vi "VI to JSON Graph Descr.vi"(8 "error in (no error)":errorcluster, 11 "vi path":path) -> (0 "error out":errorcluster, 1 "# of Refs":i32, 2 "Objects with owner":T2[](array[typedef]) {"Ownder_UID" format="%x"; "UID" format="%x"; "ClassID" format="%x"})   [LabVIEW 2020]
uses:
  ObjDescription.ctl
  Wire_Source_and_Sinks_IDs.ctl
  <vilib>/Utility/traverseref.llb/TRef TravTarget.ctl
  <vilib>/Utility/traverseref.llb/VI Scripting - Traverse.lvlib
panel:
  out "Wires":T1[](array[typedef])
  in  "Traverse Generated Code (F)":bool
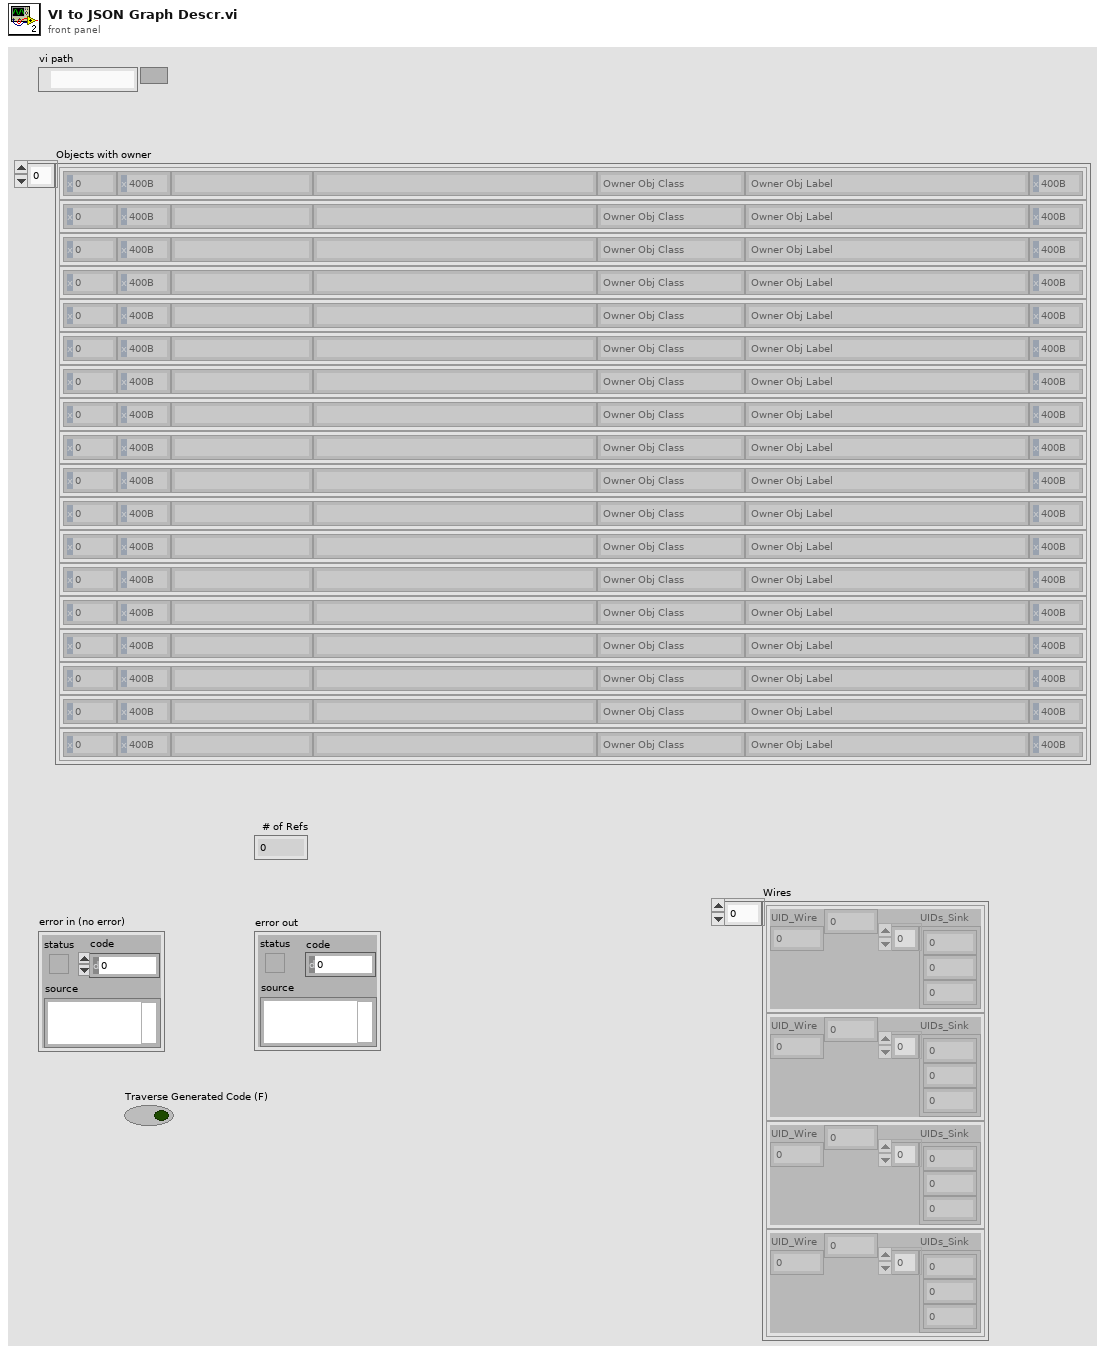
[diagram p1: front panel]
types:
  T1 = typedef "Wire_Source_and_Sinks_IDs.ctl" = cluster{"UID_Wire":i32, "UID_Source":i32, "UIDs_Sink":i32[]}
  T2 = typedef "ObjDescription.ctl" = cluster{"ClassID":u32, "UID":u32, "ClassName":string, "LabelText":string, "OwnerClass":string, "OwnerName":string, "Ownder_UID":u32}
  T3 = typedef "TRef TravTarget.ctl" = enum16{"FP", "BD", "Other"}
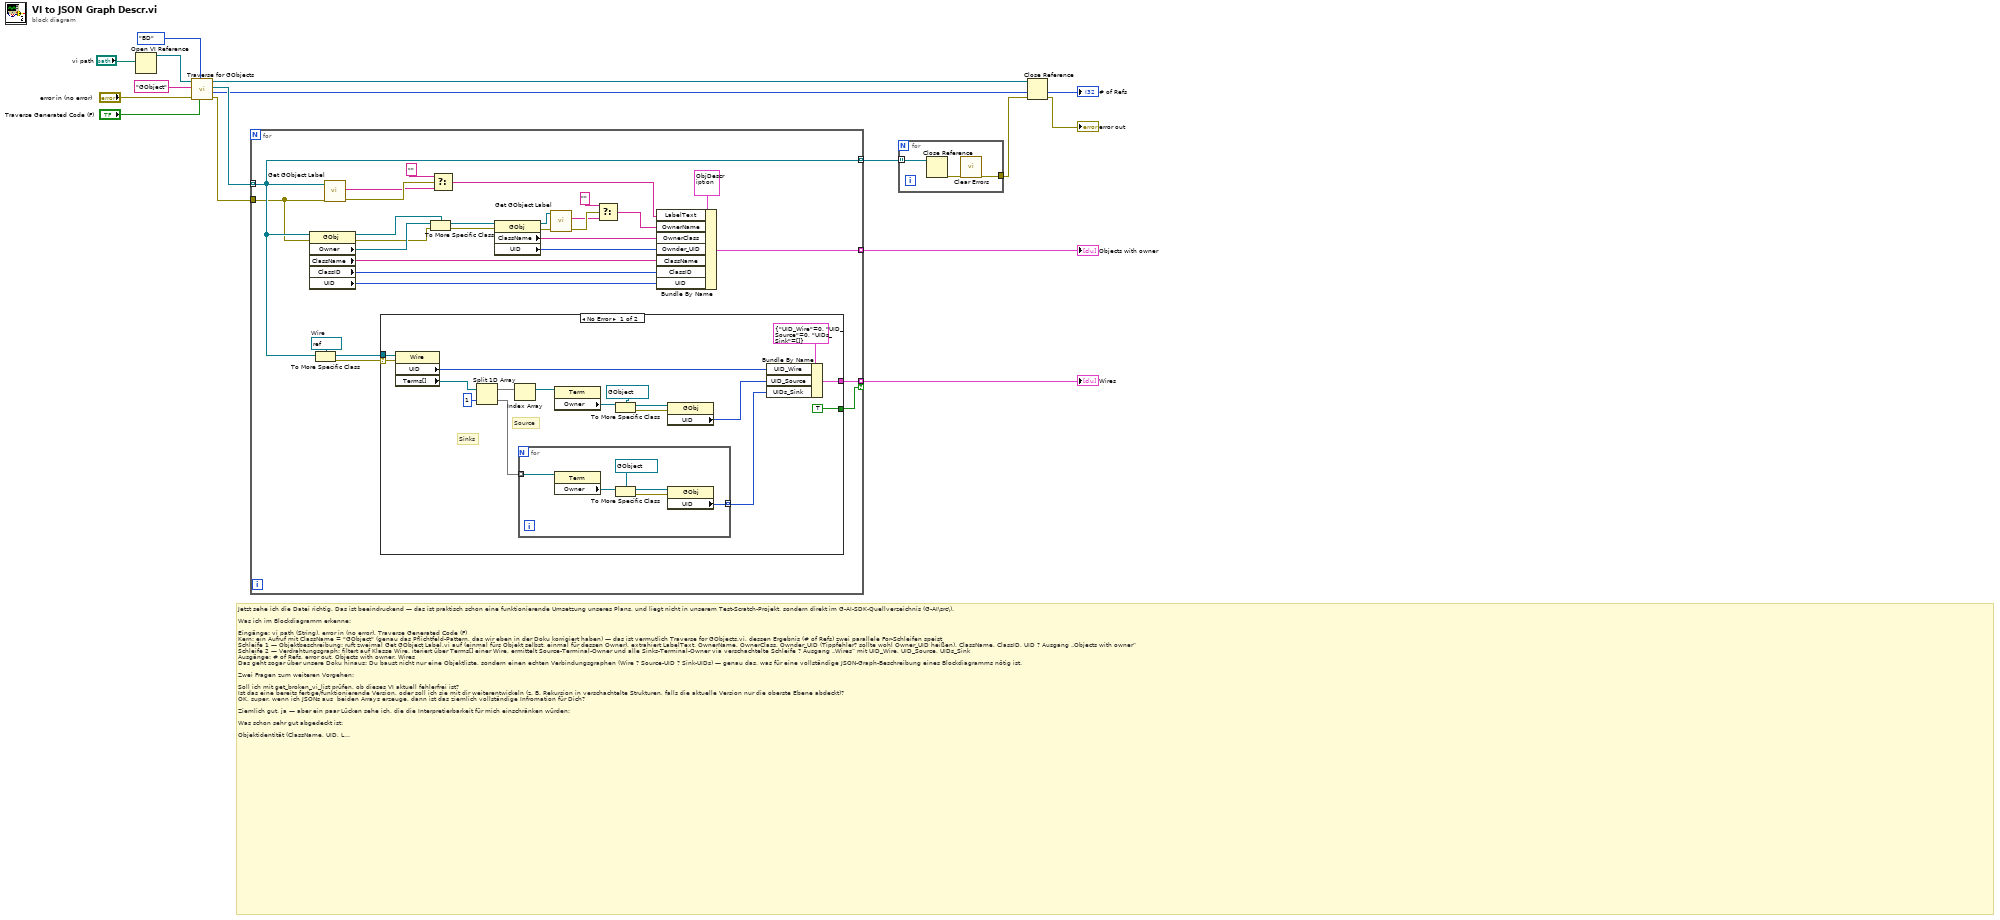
[diagram p0: block diagram]
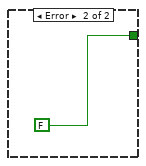
[diagram p2: hidden frame]
diagram:
  # "Jetzt sehe ich die Datei richtig. Das ist beeindruckend — das ist praktisch schon eine funktionierende Umsetzung unseres Plans, und liegt nicht in unserem Test-Scratch-Projekt, sondern direkt im G-AI-SDK-Quellverzeichnis (G-AI\\src\\).\n\nWas ich im Blockdiagramm erkenne:\n\nEingänge: vi path (String), error in (no error), Traverse Generated Code (F)\nKern: ein Aufruf mit ClassName = \"GObject\" (genau das Pflichtfeld-Pattern, das wir eben in der Doku korrigiert haben) — das ist vermutlich Traverse for GObjects.vi, dessen Ergebnis (# of Refs) zwei parallele For-Schleifen speist\nSchleife 1 — Objektbeschreibung: ruft zweimal Get GObject Label.vi auf (einmal fürs Objekt selbst, einmal für dessen Owner), extrahiert LabelText, OwnerName, OwnerClass, Ownder_UID (Tippfehler? sollte wohl Owner_UID heißen), ClassName, ClassID, UID ? Ausgang „Objects with owner“\nSchleife 2 — Verdrahtungsgraph: filtert auf Klasse Wire, iteriert über Terms[] einer Wire, ermittelt Source-Terminal-Owner und alle Sinks-Terminal-Owner via verschachtelte Schleife ? Ausgang „Wires“ mit UID_Wire, UID_Source, UIDs_Sink\nAusgänge: # of Refs, error out, Objects with owner, Wires\nDas geht sogar über unsere Doku hinaus: Du baust nicht nur eine Objektliste, sondern einen echten Verbindungsgraphen (Wire ? Source-UID ? Sink-UIDs) — genau das, was für eine vollständige JSON-Graph-Beschreibung eines Blockdiagramms nötig ist.\n\nZwei Fragen zum weiteren Vorgehen:\n\nSoll ich mit get_broken_vi_list prüfen, ob dieses VI aktuell fehlerfrei ist?\nIst das eine bereits fertige/funktionierende Version, oder soll ich sie mit dir weiterentwickeln (z. B. Rekursion in verschachtelte Strukturen, falls die aktuelle Version nur die oberste Ebene abdeckt)?\nOK, super. wenn ich JSONs aus  beiden Arrays erzeuge, dann ist das ziemlich vollständige Infromation für Dich?\n\nZiemlich gut, ja — aber ein paar Lücken sehe ich, die die Interpretierbarkeit für mich einschränken würden:\n\nWas schon sehr gut abgedeckt ist:\n\nObjektidentität (ClassName, UID, LabelText) und Eltern-Zuordnung (Owner_UID) ? daraus lässt sich die volle Verschachtelungshierarchie rekonstruieren (Objekt ? Diagramm ? Struktur ? äußeres Diagramm …), auch über mehrere Ebenen, indem man die Owner_UID-Kette verfolgt.\nGrundlegende Konnektivität (Wires: welches Objekt mit welchem verbunden ist).\nKonkrete Lücken, die ich als problematisch einschätze:\n\nTerminal-Ebene fehlt bei den Wires. UID_Source/UIDs_Sink verweisen auf den Owner des Terminals (also den Node), nicht auf das Terminal selbst. Bei Nodes mit mehreren Ein-/Ausgängen (z. B. Bundle, ein SubVI mit 5 Parametern, Add mit X/Y) kann ich dann nicht unterscheiden, welcher Eingang/Ausgang gemeint ist — nur dass irgendeine Verbindung zwischen den beiden Nodes existiert. Für echtes Datenfluss-Verständnis würde ich zusätzlich Terminal-Name oder -Index pro Wire-Ende brauchen.\nKonstanten-Werte fehlen. LabelText ist der Objekt-Label, nicht der tatsächliche Wert einer Konstante (z. B. Numeric Constant = 5). Ohne Wert sehe ich nur \"hier ist eine Zahlenkonstante\", nicht welche Rolle sie in der Logik spielt.\nCase-Struktur-Frame-Zugehörigkeit unklar. Wenn Traverse for GObjects.vi alle Frames eines Case-Structure flach durchläuft, brauche ich pro Objekt (oder pro Diagram-Objekt) den Frame-Namen, sonst sehe ich Objekte aus verschiedenen Cases undifferenziert vermischt.\nSubVI-Identität nur implizit über Label. Bei SubVI-Call-Nodes ist der Label meist automatisch der VI-Name — funktioniert praktisch meistens, ist aber nicht garantiert robust (z. B. bei umbenannten Labels).\n(nice-to-have, nicht kritisch) Bounds/Position fehlt — nur relevant, falls du auch Layout/Visualisierung rekonstruieren willst, nicht fürs reine Logikverständnis.\nWenn du 1–3 noch ergänzt, wäre das für mich praktisch vollständig nutzbar, um Datenfluss und Struktur eines VIs korrekt zu verstehen."
  n1 = Open VI Reference(vi path="vi path") -> (vi reference=w13:refnum<vi>)  [unwired: 5 in, 1 out]
  n2 = call <vilib>:"Traverse for GObjects.vi"("Traverse Generated Code (F)"="Traverse Generated Code (F)", "Traverse Target"=TRef_TravTarget."BD", "error in (no error)"="error in (no error)", "Class Name"="GObject", "VI Refnum"=w13) -> ("error out"=w4:errorcluster, "# of Refs"=→"# of Refs":i32, "References"=w15:refnum<vi>[], "dup VI Refnum"=w5:refnum<vi>)  [unwired: 3 in]
  n3 = for {
    tunnel: w15 -> [w19] mode=indexing
    tunnel: [w39] -> w12 mode=indexing
    tunnel: [w19] -> w6 mode=indexing
    tunnel: w4 -> [w18]
    tunnel: [w17] -> w3 mode=indexing if=w16
    w25 = refnum<vi> refnum  # Wire
    n4 = property class="GObj"(reference=w19, error in=w18) -> (reference out=w26:refnum<vi>, error out=w30:errorcluster, "Owner"=w42:refnum<vi>, "ClassName"=w21:string, "ClassID"=w20:u32, "UID"=w28:i32)
    n5 = To More Specific Class(target class=w25, reference=w19) -> (specific class reference=w24:refnum<vi>, error out=w23:errorcluster)  [unwired: 1 in]
    n6 = call <vilib>:"Get GObject Label.vi"("error in (no error)"=w18, "GObject"=w19) -> ("error out"=w43:errorcluster, "Object Label"=w41:string)  [unwired: 5 in, 3 out]
    n7 = case shown="No Error" w23 {
      selector: w23 -> [w60 _]
      tunnel: w24 -> [w61 _]
      tunnel: [w51 _] -> w17
      tunnel: [TRUE FALSE] -> w16
      frame No Error {
        # "Sinks"
        # "Source"
        n8 = property class="Wire"(reference=w61, error in=w60) -> ("UID"=w46:i32, "Terms[]"=w49:refnum<vi>[])  [unwired: 2 out]
        n9 = Split 1D Array(array=w49, index=1 ("length")) -> (first subarray=w57:refnum<vi>[], second subarray=w56:refnum<vi>[])
        n10 = Index Array(array=w57) -> (element=w58:refnum<vi>)  [unwired: 1 in]
        n11 = for {
          tunnel: w56 -> [w67] mode=indexing
          tunnel: [w62] -> w45 mode=indexing
          n12 = property class="Term"(reference=w67) -> ("Owner"=w63:refnum<vi>)  [unwired: 1 in, 2 out]
          n13 = To More Specific Class(target class=refnum<vi> refnum ("reference out"), reference=w63) -> (specific class reference=w65:refnum<vi>, error out=w64:errorcluster)  [unwired: 1 in]
          n14 = property class="GObj"(reference=w65, error in=w64) -> ("UID"=w62:i32)  [unwired: 2 out]
        }
        n15 = property class="Term"(reference=w58) -> ("Owner"=w53:refnum<vi>)  [unwired: 1 in, 2 out]
        n16 = To More Specific Class(target class=refnum<vi> refnum ("reference out"), reference=w53) -> (specific class reference=w54:refnum<vi>, error out=w55:errorcluster)  [unwired: 1 in]
        n17 = property class="GObj"(reference=w54, error in=w55) -> ("UID"=w47:i32)  [unwired: 2 out]
        n18 = Bundle By Name(cluster=T1 {"UID_Wire"=0, "UID_Source"=0, "UIDs_Sink"=[]} ("output cluster"), "UID_Wire"=w46, "UID_Source"=w47, "UIDs_Sink"=w45) -> (w51:T1)
      }
      frame Error {
      }
    }
    n19 = To More Specific Class(target class=w26, reference=w42, error in=w30) -> (specific class reference=w34:refnum<vi>, error out=w29:errorcluster)
    n20 = Select(t="", s=w43, f=w41) -> (s? t:f=w22:string)
    n21 = property class="GObj"(reference=w34, error in=w29) -> (reference out=w33:refnum<vi>, error out=w31:errorcluster, "ClassName"=w27:string, "UID"=w32:i32)
    n22 = call <vilib>:"Get GObject Label.vi"("error in (no error)"=w31, "GObject"=w33) -> ("error out"=w44:errorcluster, "Object Label"=w36:string)  [unwired: 5 in, 3 out]
    n23 = Select(t="", s=w44, f=w36) -> (s? t:f=w35:string)
    n24 = Bundle By Name(cluster=T2 {"ClassID"=16395, "UID"=16395, "ClassName"="ControlTerminal", "LabelText"="ControlTerminal", "OwnerClass"="Owner Obj Class", "OwnerName"="Owner Obj Label", "Ownder_UID"=16395} ("Cluster"), "LabelText"=w22, "OwnerName"=w35, "OwnerClass"=w27, "Ownder_UID"=w32, "ClassName"=w21, "ClassID"=w20, "UID"=w28) -> (w39:T2)
  }
  "Objects with owner" <- w12
  "Wires" <- w3
  n25 = for {
    tunnel: w6 -> [w71] mode=indexing
    tunnel: [w69] -> w2
    n26 = Close Reference(reference=w71) -> (error out=w70:errorcluster)  [unwired: 1 in]
    n27 = call <vilib>:"Clear Errors.vi"("error in (no error)"=w70) -> ("error out"=w69:errorcluster)  [unwired: 5 in, 1 out]
  }
  n28 = Close Reference(reference=w5, error in (no error)=w2) -> (error out=→"error out":errorcluster)
